vi "Save Raw Data.vi"(8 "error in (no error)":errorcluster, 10 "Raw Data Results":T2={"BW 1 Resistance"="0.7817\n", "BW 2 Resistance"="1.2990\n", "No-Fire Results BW1"={"Current"=["7.203409E-06\n", "7.484487E-06\n", "7.484465E-06\n", "8.327806E-06\n", "7.765564E-06\n", "7.062867E-06\n", "8.187235E-06\n", "8.187257E-06\n", "7.906143E-06\n", "7.765622E-06\n", "7.203482E-06\n", "7.484487E-06\n", "7.484487E-06\n", "7.625029E-06\n", "7.765600E-06\n", "7.203387E-06\n", "7.625014E-06\n", "7.765651E-06\n", "8.046671E-06\n", "7.906223E-06\n", "7.343981E-06\n", "7.203409E-06\n", "7.625109E-06\n", "7.765608E-06\n", "7.906143E-06\n", "8.187286E-06\n", "8.046729E-06\n", "7.484501E-06\n", "8.046707E-06\n", "7.906157E-06\n", "7.484501E-06\n", "7.062881E-06\n", "7.906165E-06\n", "7.625087E-06\n", "7.906179E-06\n", "7.765622E-06\n", "7.765593E-06\n", "7.343951E-06\n", "7.906230E-06\n", "7.625087E-06\n", "7.062867E-06\n", "7.484530E-06\n", "7.906172E-06\n", "7.906157E-06\n", "7.625029E-06\n", "7.906143E-06\n", "7.625073E-06\n", "7.343959E-06\n", "8.187249E-06\n", "8.187220E-06\n", "8.187286E-06\n", "7.906172E-06\n", "7.484487E-06\n", "7.765608E-06\n", "7.625073E-06\n", "7.906172E-06\n", "7.906179E-06\n", "7.484523E-06\n", "7.625051E-06\n", "7.765593E-06\n", "7.484559E-06\n", "7.765637E-06\n", "7.484581E-06\n", "8.046714E-06\n", "7.765630E-06\n", "7.765651E-06\n", "8.187286E-06\n", "8.046707E-06\n", "7.906143E-06\n", "8.046729E-06\n", "7.906143E-06\n", "8.046773E-06\n", "7.625065E-06\n", "7.344046E-06\n", "8.327836E-06\n", "7.765644E-06\n", "7.765630E-06\n", "7.484545E-06\n", "7.765615E-06\n", "7.765644E-06\n", "7.203424E-06\n", "7.906143E-06\n", "7.484523E-06\n", "8.046758E-06\n", "7.765666E-06\n", "7.906165E-06\n", "7.625073E-06\n", "8.327777E-06\n", "7.484523E-06\n", "7.625073E-06\n", "7.906150E-06\n", "7.625065E-06\n", "7.625065E-06\n", "7.765630E-06\n", "7.625124E-06\n", "7.765615E-06\n", "7.484494E-06\n", "7.343966E-06\n", "7.906216E-06\n", "7.765608E-06\n", "7.906194E-06\n", "7.484581E-06\n", "7.765622E-06\n", "7.906208E-06\n", "7.343973E-06\n", "7.062918E-06\n", "7.343981E-06\n", "7.765579E-06\n", "7.484530E-06\n", "7.765637E-06\n", "7.625087E-06\n", "8.046707E-06\n", "8.468349E-06\n", "7.906179E-06\n", "7.625065E-06\n", "7.906150E-06\n", "7.906194E-06\n", "7.765644E-06\n", "7.765622E-06\n", "8.187257E-06\n", "7.484501E-06\n", "7.765608E-06\n", "7.343973E-06\n", "7.906143E-06\n", "7.625051E-06\n", "7.906150E-06\n", "7.765593E-06\n", "7.625044E-06\n", "7.765622E-06\n", "7.625102E-06\n", "7.343959E-06\n", "7.484588E-06\n", "7.765622E-06\n", "7.625109E-06\n", "7.906172E-06\n", "7.343973E-06\n", "7.625102E-06\n", "8.468385E-06\n", "7.906201E-06\n", "7.906194E-06\n", "8.046707E-06\n", "7.625109E-06\n", "7.906172E-06\n", "7.906179E-06\n", "8.046773E-06\n", "7.906216E-06\n", "8.327799E-06\n", "7.906223E-06\n", "7.343995E-06\n", "8.046714E-06\n", "8.046685E-06\n"], "Voltage"=[], "Time"=[]}, "No-Fire Results BW2"={"Current"=["7.203409E-06\n", "7.484487E-06\n", "7.484465E-06\n", "8.327806E-06\n", "7.765564E-06\n", "7.062867E-06\n", "8.187235E-06\n", "8.187257E-06\n", "7.906143E-06\n", "7.765622E-06\n", "7.203482E-06\n", "7.484487E-06\n", "7.484487E-06\n", "7.625029E-06\n", "7.765600E-06\n", "7.203387E-06\n", "7.625014E-06\n", "7.765651E-06\n", "8.046671E-06\n", "7.906223E-06\n", "7.343981E-06\n", "7.203409E-06\n", "7.625109E-06\n", "7.765608E-06\n", "7.906143E-06\n", "8.187286E-06\n", "8.046729E-06\n", "7.484501E-06\n", "8.046707E-06\n", "7.906157E-06\n", "7.484501E-06\n", "7.062881E-06\n", "7.906165E-06\n", "7.625087E-06\n", "7.906179E-06\n", "7.765622E-06\n", "7.765593E-06\n", "7.343951E-06\n", "7.906230E-06\n", "7.625087E-06\n", "7.062867E-06\n", "7.484530E-06\n", "7.906172E-06\n", "7.906157E-06\n", "7.625029E-06\n", "7.906143E-06\n", "7.625073E-06\n", "7.343959E-06\n", "8.187249E-06\n", "8.187220E-06\n", "8.187286E-06\n", "7.906172E-06\n", "7.484487E-06\n", "7.765608E-06\n", "7.625073E-06\n", "7.906172E-06\n", "7.906179E-06\n", "7.484523E-06\n", "7.625051E-06\n", "7.765593E-06\n", "7.484559E-06\n", "7.765637E-06\n", "7.484581E-06\n", "8.046714E-06\n", "7.765630E-06\n", "7.765651E-06\n", "8.187286E-06\n", "8.046707E-06\n", "7.906143E-06\n", "8.046729E-06\n", "7.906143E-06\n", "8.046773E-06\n", "7.625065E-06\n", "7.344046E-06\n", "8.327836E-06\n", "7.765644E-06\n", "7.765630E-06\n", "7.484545E-06\n", "7.765615E-06\n", "7.765644E-06\n", "7.203424E-06\n", "7.906143E-06\n", "7.484523E-06\n", "8.046758E-06\n", "7.765666E-06\n", "7.906165E-06\n", "7.625073E-06\n", "8.327777E-06\n", "7.484523E-06\n", "7.625073E-06\n", "7.906150E-06\n", "7.625065E-06\n", "7.625065E-06\n", "7.765630E-06\n", "7.625124E-06\n", "7.765615E-06\n", "7.484494E-06\n", "7.343966E-06\n", "7.906216E-06\n", "7.765608E-06\n", "7.906194E-06\n", "7.484581E-06\n", "7.765622E-06\n", "7.906208E-06\n", "7.343973E-06\n", "7.062918E-06\n", "7.343981E-06\n", "7.765579E-06\n", "7.484530E-06\n", "7.765637E-06\n", "7.625087E-06\n", "8.046707E-06\n", "8.468349E-06\n", "7.906179E-06\n", "7.625065E-06\n", "7.906150E-06\n", "7.906194E-06\n", "7.765644E-06\n", "7.765622E-06\n", "8.187257E-06\n", "7.484501E-06\n", "7.765608E-06\n", "7.343973E-06\n", "7.906143E-06\n", "7.625051E-06\n", "7.906150E-06\n", "7.765593E-06\n", "7.625044E-06\n", "7.765622E-06\n", "7.625102E-06\n", "7.343959E-06\n", "7.484588E-06\n", "7.765622E-06\n", "7.625109E-06\n", "7.906172E-06\n", "7.343973E-06\n", "7.625102E-06\n", "8.468385E-06\n", "7.906201E-06\n", "7.906194E-06\n", "8.046707E-06\n", "7.625109E-06\n", "7.906172E-06\n", "7.906179E-06\n", "8.046773E-06\n", "7.906216E-06\n", "8.327799E-06\n", "7.906223E-06\n", "7.343995E-06\n", "8.046714E-06\n", "8.046685E-06\n"], "Voltage"=[], "Time"=[]}, "ACW Results BW1"={"ACW Time BW1"=[], "ACW Voltage BW1"=[], "ACW Current BW1"=[]}, "IR Results BW1"={"Max Leakage Current (A)"=0.0, "Min Leakage Current (A)"=0.0, "Max Change in Current (A)"=0.0, "Dielectric Strength Pass?"=FALSE, "Insulation Resistance Pass?"=FALSE, "Insulation Resistance"=""}, "ACW Results BW2"={"ACW Time BW2"=[], "ACW Voltage BW2"=[], "ACW Current BW2"=[]}, "IR Results BW 2"={"Max Leakage Current (A)"=0.0, "Min Leakage Current (A)"=0.0, "Max Change in Current (A)"=0.0, "Dielectric Strength Pass?"=FALSE, "Insulation Resistance Pass?"=FALSE, "Insulation Resistance"=""}}, 11 "file path (dialog if empty)":path) -> (0 "error out":errorcluster)   [LabVIEW 2018]
uses:
  <vilib>/Utility/file.llb/Write Delimited Spreadsheet (string).vi
panel:
  in  "BW 2 Results 2":T1
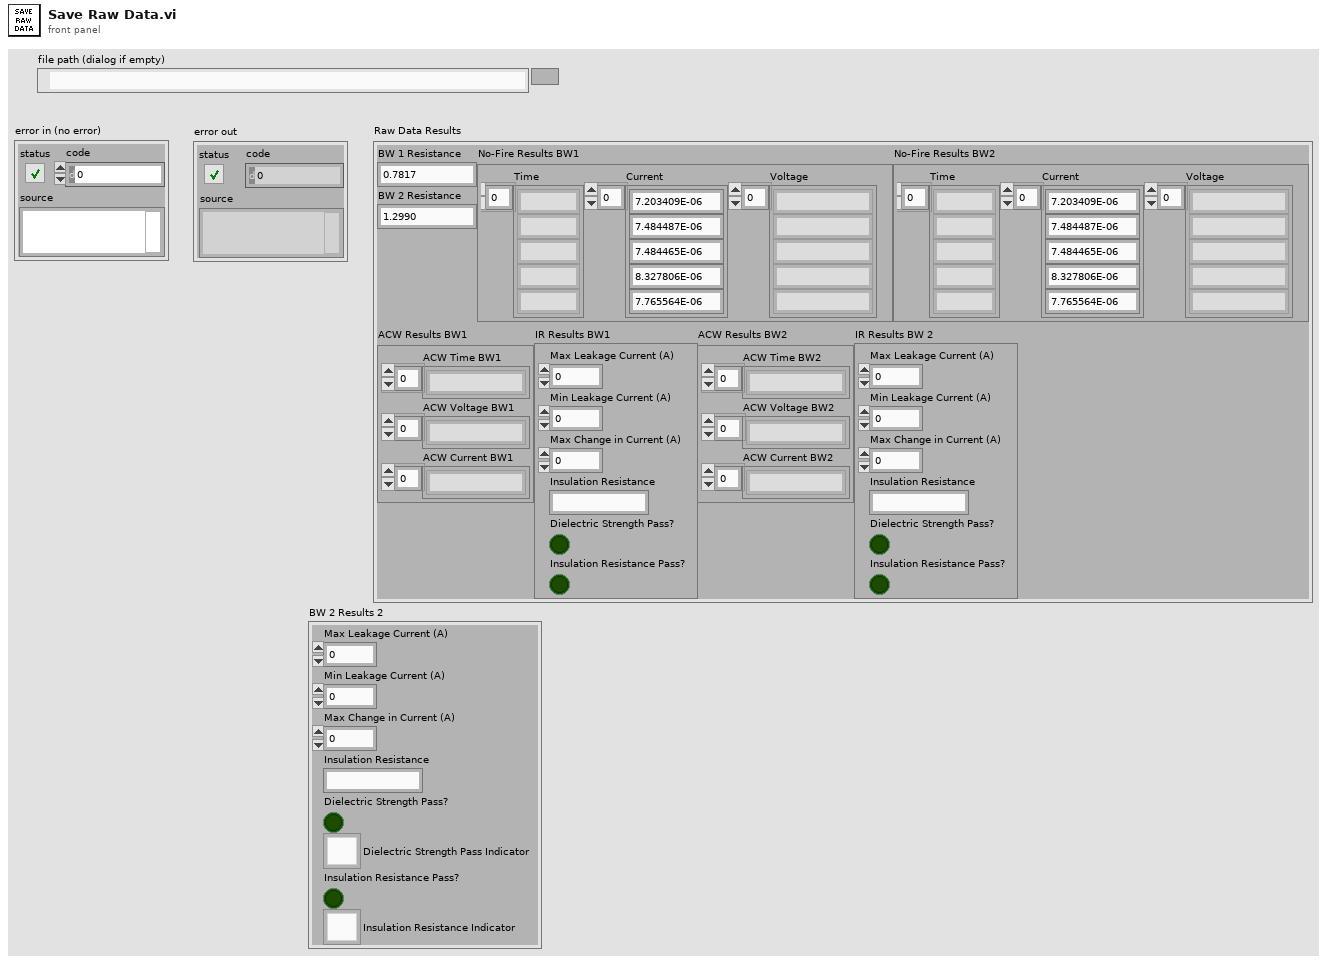
[diagram p1: front panel]
types:
  T1 = cluster{"Max Leakage Current (A)":dbl, "Min Leakage Current (A)":dbl, "Max Change in Current (A)":dbl, "Dielectric Strength Pass?":bool, "Insulation Resistance Pass?":bool, "Insulation Resistance":string, "Dielectric Strength Pass Indicator":u16, "Insulation Resistance Indicator":u16}
  T2 = cluster{"BW 1 Resistance":string, "BW 2 Resistance":string, "No-Fire Results BW1":cluster{"Current":string[], "Voltage":string[], "Time":string[]}, "No-Fire Results BW2":cluster{"Current":string[], "Voltage":string[], "Time":string[]}, "ACW Results BW1":cluster{"ACW Time BW1":string[], "ACW Voltage BW1":string[], "ACW Current BW1":string[]}, "IR Results BW1":cluster{"Max Leakage Current (A)":dbl, "Min Leakage Current (A)":dbl, "Max Change in Current (A)":dbl, "Dielectric Strength Pass?":bool, "Insulation Resistance Pass?":bool, "Insulation Resistance":string}, "ACW Results BW2":cluster{"ACW Time BW2":string[], "ACW Voltage BW2":string[], "ACW Current BW2":string[]}, "IR Results BW 2":cluster{"Max Leakage Current (A)":dbl, "Min Leakage Current (A)":dbl, "Max Change in Current (A)":dbl, "Dielectric Strength Pass?":bool, "Insulation Resistance Pass?":bool, "Insulation Resistance":string}}
  T3 = cluster{"Current":string[], "Voltage":string[], "Time":string[]}
  T4 = cluster{"ACW Time BW1":string[], "ACW Voltage BW1":string[], "ACW Current BW1":string[]}
  T5 = cluster{"Max Leakage Current (A)":dbl, "Min Leakage Current (A)":dbl, "Max Change in Current (A)":dbl, "Dielectric Strength Pass?":bool, "Insulation Resistance Pass?":bool, "Insulation Resistance":string}
  T6 = cluster{"ACW Time BW2":string[], "ACW Voltage BW2":string[], "ACW Current BW2":string[]}
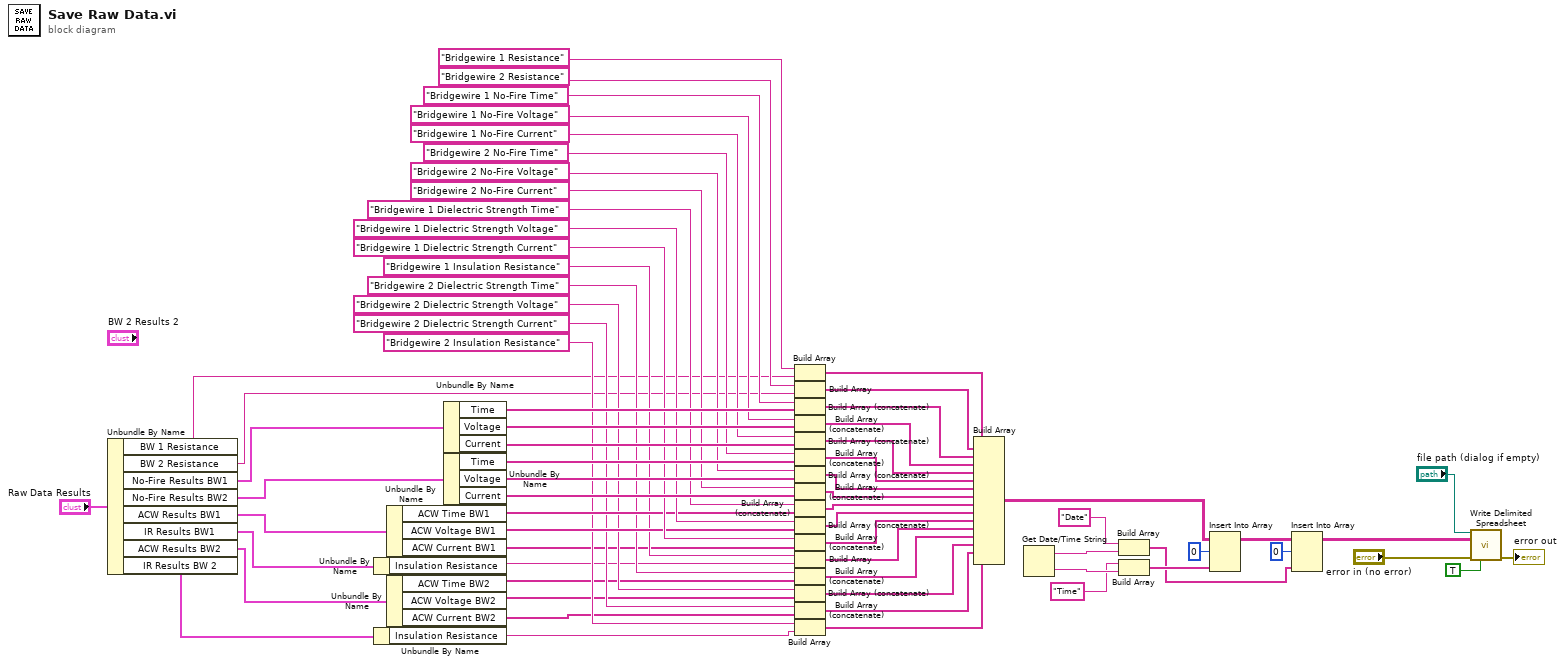
[diagram p0: block diagram]
diagram:
  n1 = Unbundle By Name("Raw Data Results") -> ("BW 1 Resistance"=w17:string, "BW 2 Resistance"=w16:string, "No-Fire Results BW1"=w23:T3, "No-Fire Results BW2"=w22:T3, "ACW Results BW1"=w21:T4, "IR Results BW1"=w20:T5, "ACW Results BW2"=w19:T6, "IR Results BW 2"=w18:T5)
  n2 = Unbundle By Name(w20) -> ("Insulation Resistance"=w42:string)
  n3 = Unbundle By Name(w18) -> ("Insulation Resistance"=w38:string)
  n4 = Unbundle By Name(w21) -> ("ACW Time BW1"=w50:string[], "ACW Voltage BW1"=w49:string[], "ACW Current BW1"=w43:string[])
  n5 = Unbundle By Name(w19) -> ("ACW Time BW2"=w41:string[], "ACW Voltage BW2"=w40:string[], "ACW Current BW2"=w39:string[])
  n6 = Unbundle By Name(w23) -> ("Time"=w64:string[], "Voltage"=w63:string[], "Current"=w61:string[])
  n7 = Unbundle By Name(w22) -> ("Time"=w59:string[], "Voltage"=w57:string[], "Current"=w55:string[])
  n8 = Build Array("Bridgewire 1 Resistance" ("element"), w17) -> (w69:string[])
  n9 = Build Array("Bridgewire 2 Resistance" ("element"), w16) -> (w70:string[])
  n10 = Build Array (concatenate)("Bridgewire 1 No-Fire Time" ("element"), w64) -> (w66:string[])
  n11 = Build Array (concatenate)("Bridgewire 1 No-Fire Voltage" ("element"), w63) -> (w37:string[])
  n12 = Build Array (concatenate)("Bridgewire 1 No-Fire Current" ("element"), w61) -> (w36:string[])
  n13 = Build Array (concatenate)("Bridgewire 2 No-Fire Time" ("element"), w59) -> (w35:string[])
  n14 = Build Array (concatenate)("Bridgewire 2 No-Fire Voltage" ("element"), w57) -> (w34:string[])
  n15 = Build Array (concatenate)("Bridgewire 2 No-Fire Current" ("element"), w55) -> (w33:string[])
  n16 = Build Array (concatenate)("Bridgewire 1 Dielectric Strength Time" ("element"), w50) -> (w32:string[])
  n17 = Build Array (concatenate)("Bridgewire 1 Dielectric Strength Voltage" ("element"), w49) -> (w31:string[])
  n18 = Build Array (concatenate)("Bridgewire 1 Dielectric Strength Current" ("element"), w43) -> (w30:string[])
  n19 = Build Array("Bridgewire 1 Insulation Resistance" ("element"), w42) -> (w29:string[])
  n20 = Build Array (concatenate)("Bridgewire 2 Dielectric Strength Time" ("element"), w41) -> (w28:string[])
  n21 = Build Array (concatenate)("Bridgewire 2 Dielectric Strength Voltage" ("element"), w40) -> (w27:string[])
  n22 = Build Array (concatenate)("Bridgewire 2 Dielectric Strength Current" ("element"), w39) -> (w26:string[])
  n23 = Build Array("Bridgewire 2 Insulation Resistance" ("element"), w38) -> (w25:string[])
  n24 = Build Array(w69, w70, w66, w37, w36, w35, w34, w33, w32, w31, w30, w29, w28, w27, w26, w25) -> (w15:string[][])
  n25 = Get Date/Time String() -> (date string=w7:string, time string=w13:string)  [unwired: 3 in]
  n26 = Build Array("Date" ("element"), w7) -> (w6:string[])
  n27 = Build Array("Time" ("element"), w13) -> (w12:string[])
  n28 = Insert Into Array(array=w15, index (row)=0, new element=w12) -> (w10:string[][])  [unwired: 1 in]
  n29 = Insert Into Array(array=w10, index (row)=0, new element=w6) -> (w1:string[][])  [unwired: 1 in]
  n30 = call-poly <vilib>:"Write Delimited Spreadsheet.vi"("file path (dialog if empty)"="file path (dialog if empty)", "2D data"=w1, "error in (no error)"="error in (no error)", "transpose? (no:F)"=TRUE) -> ("error out"=→"error out":errorcluster)  [unwired: 10 in, 1 out]
